vi "Begin.vi"(8 "error in":errorcluster) -> (0 "error out":errorcluster)   [LabVIEW 2014]
doc: "Called before other user functions, this VI is expected to open initial I/O refnums, load in file data, and do all program initialization. Notice that the <B>error out</B> terminal is simply used for data flow. Wiring it to other structures or subVIs ensures that this VI runs first."
uses:
  <vilib>/Rock Robotics/WPI/DriverStation/WPI_DriverStationRobotMode2.ctl
  Global Variables.vi
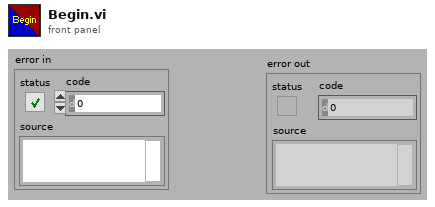
[diagram p1: front panel]
types:
  T1 = typedef "WPI_DriverStationRobotMode2.ctl" = enum16{"Autonomous Disabled", "Autonomous Enabled", "Teleop Disabled", "Teleop Enabled", "Disconnected", "Finish", "Test Disabled", "Test Enabled", "Emergency Stopped"}
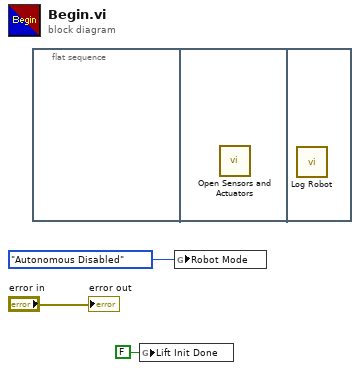
[diagram p0: block diagram]
diagram:
  n1 = flat-sequence {
    frame #0 {
    }
    frame #1 {
      n2 = call "Open Sensors and Actuators.vi"() -> ()  [unwired: 12 in]
    }
    frame #2 {
      n3 = call "Log Robot.vi"() -> ()  [unwired: 12 in]
    }
  }
  n4 = global write "Global Variables.vi" "Lift Init Done"(FALSE ("Lift Init Done")) -> ()
  n5 = global write "Global Variables.vi" "Robot Mode"(WPI_DriverStationRobotMode2."Autonomous Disabled" ("Robot Mode")) -> ()
  "error out" <- "error in"
